vi "LabJackT7.vi"(4 "Scan Period":dbl format="%.2f", 5 "Previous Scan Value":dbl format="%.2f", 6 "Present scan array":dbl[](array[numeric]) format="%.2f", 7 "Value to Output":dbl format="%.2f", 8 "Ch Description":T1={"Ch Name"="", "Type"="", "Function"=enum."Analogue Input", "Ch State"=enum."On", "Calibration type"=enum."Raw", "A"=0.0, "B"=0.0, "C"=0.0, "D"=0.0, "Comments"="", "Address"={"Main"=0, "Ch."=0, "Sub"=0, "Port Name"=""}, "String"="", "Duty"=65535} {"Duty" format="%.0b"; "D" format="%#_5g"; "C" format="%#_5g"; "B" format="%#_5g"; "A" format="%#_5g"}, 9 "Ch names":string[](array[string])) -> (0 "Scan comment":string, 1 "Output":dbl format="%.7f")   [LabVIEW 2015]
uses:
  ADAM Client/Sub VIs/ADAM Controls/Ch_description_ADAM.ctl
  ADAM Client/Sub VIs/ADAM Controls/Module_type_ADAM.ctl
  ADAM Client/Sub VIs/ADAM Controls/Function_ADAM.ctl
  ADAM Client/Sub VIs/ADAM Controls/Channel_State.ctl
  ADAM Client/Sub VIs/ADAM Controls/Calib_type_ADAM.ctl
  ADAM Client/Sub VIs/ADAM Controls/Address.ctl
  ADAM Client/Sub VIs/ADAM Controls/Remember_value_mode.ctl
  <vilib>/Utility/error.llb/DialogType.ctl
panel:
  in  "MaxAge(s)":dbl=1.5
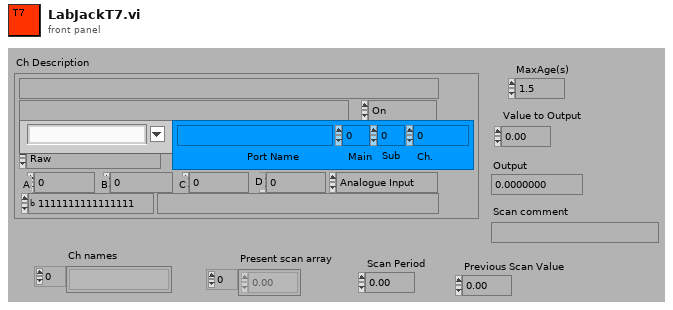
[diagram p1: front panel]
types:
  T1 = typedef "Ch_description_ADAM.ctl" = cluster{"Ch Name":string, "Type":T2, "Function":T3, "Ch State":T4, "Calibration type":T5, "A":dbl, "B":dbl, "C":dbl, "D":dbl, "Comments":string, "Address":T6, "String":string, "Duty":u16}
  T2 = typedef "Module_type_ADAM.ctl" = string
  T3 = typedef "Function_ADAM.ctl" = enum16{"Analogue Input", "Digital Input", "Event counter", "Event rate", "Analogue Output", "Digital Output", "Relay Output"}
  T4 = typedef "Channel_State.ctl" = enum16{"On", "Off", "Always On", "Always Off"}
  T5 = typedef "Calib_type_ADAM.ctl" = enum16{"Raw", "Bx + A", "Cx^2 + Bx + A", "Dx^3 + Cx^2 + Bx + A", "In Band", "Hi-Tec Q", "Hi-Tec M_dot", "Text"}
  T6 = typedef "Address.ctl" = cluster{"Main":i32, "Ch.":i32, "Sub":i32, "Port Name":string}
  T7 = typedef "Remember_value_mode.ctl" = enum16{"Read only", "Read and Write"}
  T8 = typedef "DialogType.ctl" = u16
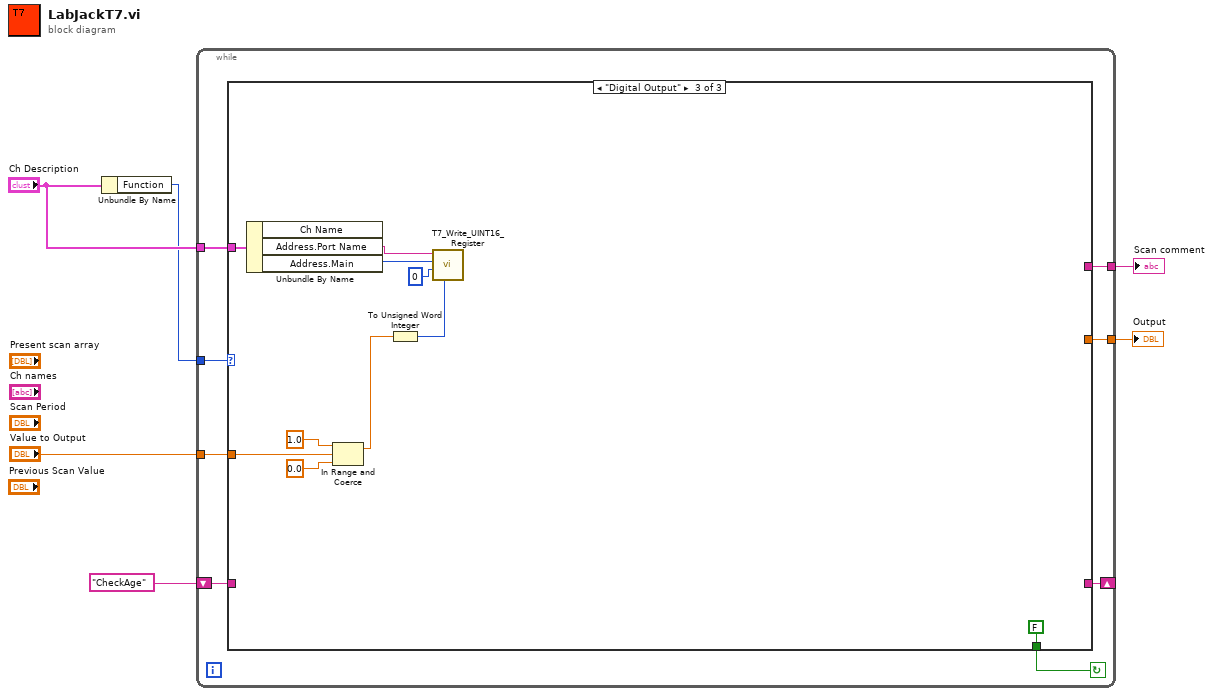
[diagram p0: block diagram]
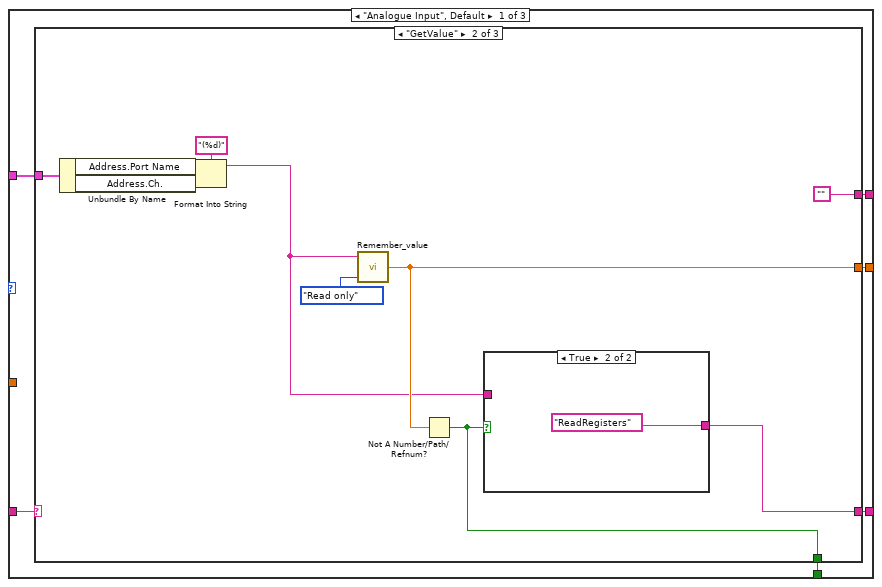
[diagram p2: hidden frame]
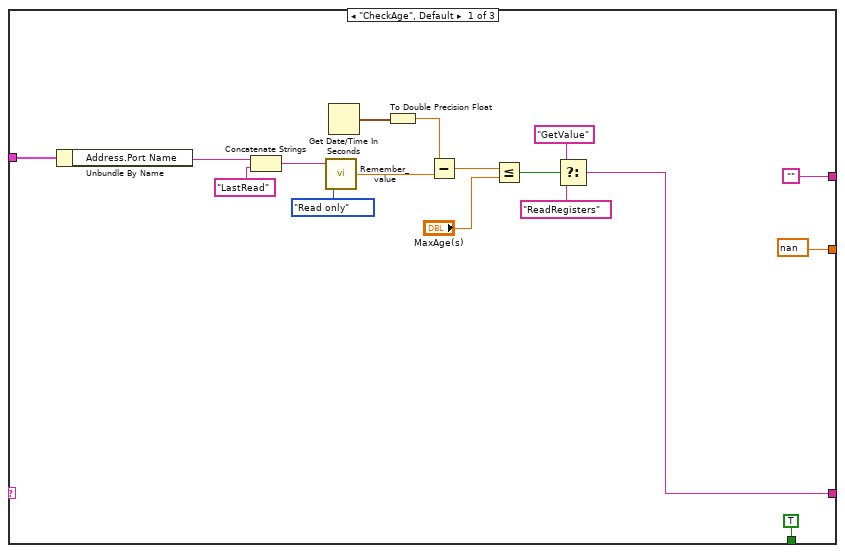
[diagram p3: hidden frame]
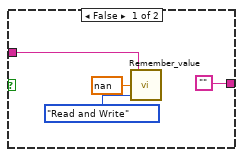
[diagram p4: hidden frame]
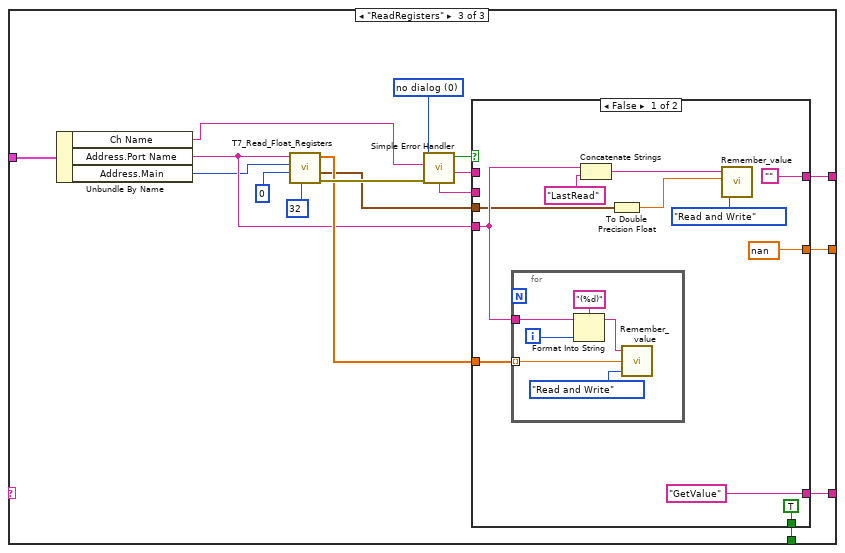
[diagram p5: hidden frame]
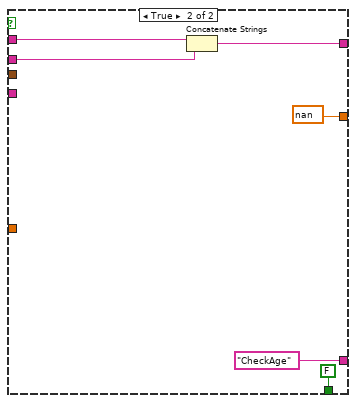
[diagram p6: hidden frame]
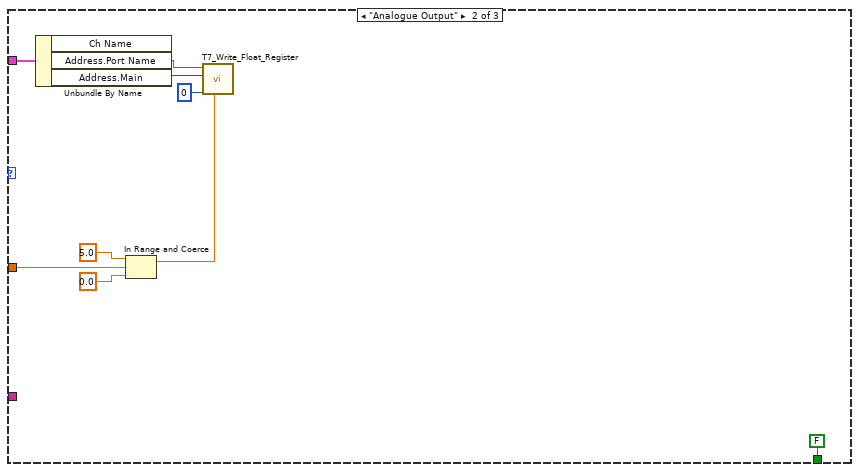
[diagram p7: hidden frame]
diagram:
  n1 = Unbundle By Name("Ch Description") -> ("Function"=w2:T3)
  n2 = while {
    tunnel: "Ch Description" -> [w14]
    tunnel: [w13] -> w6
    shift-right: [w11] -> _
    shift-left: "CheckAge" -> [w12]
    tunnel: [w9] -> w4
    tunnel: w2 -> [w8]
    tunnel: "Value to Output" -> [w7]
    stop <- w10 continue-if-true
    n3 = case shown="\"Digital Output\"" w8 {
      tunnel: w14 -> [w20 w101 w109]
      tunnel: [w19 _ _] -> w13
      tunnel: w12 -> [w18 _ _]
      tunnel: [w17 _ _] -> w11
      tunnel: [w16 FALSE FALSE] -> w10
      tunnel: [w15 _ _] -> w9
      tunnel: w7 -> [_ w96 w108]
      frame "Analogue Input", Default {
        n4 = case shown="\"GetValue\"" w18 {
          tunnel: w20 -> [w34 w47 w69]
          tunnel: ["" "" w63] -> w19
          tunnel: [w24 w40 w57] -> w17
          tunnel: [TRUE w39 w54] -> w16
          tunnel: [nan w42 w53] -> w15
          frame "CheckAge", Default {
            n5 = Unbundle By Name(w34) -> ("Address.Port Name"=w33:string)
            n6 = Concatenate Strings(w33, "LastRead" ("string")) -> (w37:string)
            n7 = call "Remember_value.vi"("Mode"=Remember_value_mode."Read only", "Ch name"=w37) -> ("Output Value"=w30:dbl)  [unwired: 1 in]
            n8 = Get Date/Time In Seconds() -> (seconds since 1Jan1904=w32:timestamp)
            n9 = To Double Precision Float(number=w32) -> (double precision float=w31:dbl)
            n10 = Subtract(x=w31, y=w30) -> (x-y=w29:dbl)
            n11 = Less Or Equal?(x=w29, y="MaxAge(s)") -> (x <= y?=w27:bool)
            n12 = Select(t="GetValue", s=w27, f="ReadRegisters") -> (s? t:f=w24:string)
          }
          frame "GetValue" {
            n13 = Unbundle By Name(w47) -> ("Address.Port Name"=w43:string, "Address.Ch."=w44:i32)
            n14 = Format Into String(format string="(%d)", initial string=w43, w44) -> (resulting string=w38:string)  [unwired: 1 in, 1 out]
            n15 = call "Remember_value.vi"("Mode"=Remember_value_mode."Read only", "Ch name"=w38) -> ("Output Value"=w42:dbl)  [unwired: 1 in]
            n16 = Not A Number/Path/Refnum?(number/path/refnum=w42) -> (NaN/Path/Refnum?=w39:bool)
            n17 = case shown="True" w39 {
              tunnel: ["" "ReadRegisters"] -> w40
              tunnel: w38 -> [w50 _]
              frame False {
                n18 = call "Remember_value.vi"("Mode"=Remember_value_mode."Read and Write", "Input Value"=nan, "Ch name"=w50) -> ()  [unwired: 1 out]
              }
              frame True {
              }
            }
          }
          frame "ReadRegisters" {
            w68 = T8 0 items=["no dialog", "OK message", "continue or stop message", "OK message + warnings", "continue/stop + warnings"] ("type of dialog (OK msg:1)")
            n19 = Unbundle By Name(w69) -> ("Ch Name"=w65:string, "Address.Port Name"=w56:string, "Address.Main"=w55:i32)
            n20 = call "T7_Read_Float_Registers.vi"("Num Registers"=u16 32, "FirstChannel"=u16 0 ("Starting Address"), "Remote Port"=w55, "Remote IP Address"=w56) -> ("error out"=w62:errorcluster, "ReadAt"=w58:timestamp, "Array"=w59:dbl[])  [unwired: 4 in, 1 out]
            n21 = call <vilib>:"Simple Error Handler.vi"("error source (\" \")"=w65, "type of dialog (OK msg:1)"=w68, "error in (no error)"=w62) -> ("error?"=w64:bool, "source out"=w66:string, "message"=w67:string)  [unwired: 4 out]
            n22 = case shown="False" w64 {
              tunnel: w67 -> [_ w91]
              tunnel: w66 -> [_ w92]
              tunnel: ["" w90] -> w63
              tunnel: w56 -> [w76 _]
              tunnel: w59 -> [w75 _]
              tunnel: w58 -> [w74 _]
              tunnel: ["GetValue" "CheckAge"] -> w57
              tunnel: [TRUE FALSE] -> w54
              tunnel: [nan nan] -> w53
              frame False {
                n23 = for {
                  tunnel: w75 -> [w86] mode=indexing
                  tunnel: w76 -> [w85]
                  i -> [w81]
                  n24 = Format Into String(format string="(%d)", initial string=w85, w81) -> (resulting string=w84:string)  [unwired: 1 in, 1 out]
                  n25 = call "Remember_value.vi"("Mode"=Remember_value_mode."Read and Write", "Input Value"=w86, "Ch name"=w84) -> ()  [unwired: 1 out]
                }
                n26 = Concatenate Strings(w76, "LastRead" ("string")) -> (w79:string)
                n27 = To Double Precision Float(number=w74) -> (double precision float=w73:dbl)
                n28 = call "Remember_value.vi"("Mode"=Remember_value_mode."Read and Write", "Input Value"=w73, "Ch name"=w79) -> ()  [unwired: 1 out]
              }
              frame True {
                n29 = Concatenate Strings(w92, w91) -> (w90:string)
              }
            }
          }
        }
      }
      frame "Analogue Output" {
        n30 = Unbundle By Name(w101) -> ("Address.Port Name"=w93:string, "Address.Main"=w100:i32)  [unwired: 1 out]
        n31 = In Range and Coerce(upper limit=5.0, x=w96, lower limit=0.0) -> (coerced(x)=w95:dbl)  [unwired: 1 out]
        n32 = call "T7_Write_Float_Register.vi"("Remote IP Address"=w93, "Remote Port"=w100, "FirstChannel"=u16 0, "FLOAT32 to Write"=w95) -> ()  [unwired: 5 in, 2 out]
      }
      frame "Digital Output" {
        n33 = Unbundle By Name(w109) -> ("Address.Port Name"=w102:string, "Address.Main"=w111:i32)  [unwired: 1 out]
        n34 = In Range and Coerce(upper limit=1.0, x=w108, lower limit=0.0) -> (coerced(x)=w105:dbl)  [unwired: 1 out]
        n35 = To Unsigned Word Integer(number=w105) -> (unsigned 16bit integer=w104:u16)
        n36 = call "T7_Write_UINT16_Register.vi"("Remote IP Address"=w102, "Remote Port"=w111, "FirstChannel"=u16 0, "UINT16 to Write"=w104) -> ()  [unwired: 5 in, 2 out]
      }
    }
  }
  "Output" <- w4
  "Scan comment" <- w6
